vi "Init.vi"(8 "error in (no error)":errorcluster, 10 "Size":cluster{"Width":u16, "Height":u16}, 11 "Glyph Drawer in":refnum<class "Glyph Drawer.lvclass">) -> (0 "error out":errorcluster, 3 "Glyph Drawer out":refnum<class "Glyph Drawer.lvclass">)   [LabVIEW 2020, in "Glyph Drawer.lvlib" / "Glyph Drawer.lvclass"]
uses:
  Glyph Drawer.lvclass
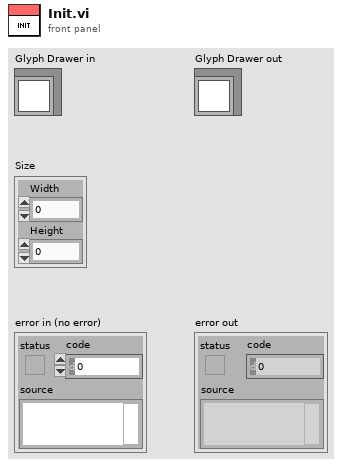
[diagram p1: front panel]
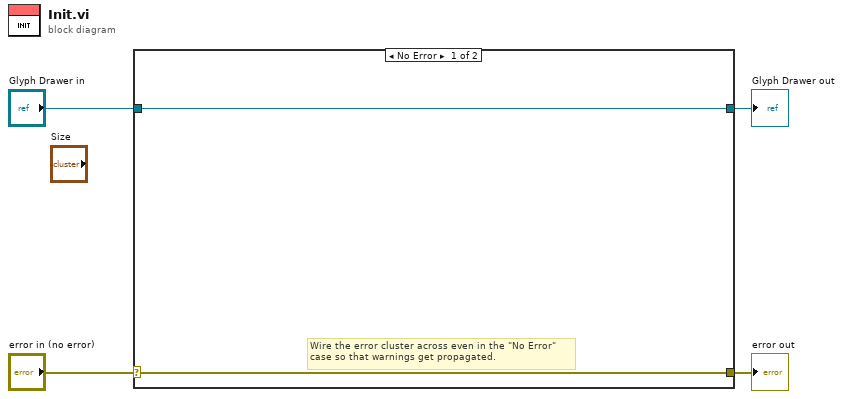
[diagram p0: block diagram]
diagram:
  n1 = case shown="No Error" "error in (no error)" {
    selector: "error in (no error)" -> [w5 w8]
    tunnel: [w5 w8] -> w3
    tunnel: [w6 w7] -> w1
    tunnel: "Glyph Drawer in" -> [w6 w7]
    frame No Error {
      # "Wire the error cluster across even in the \"No Error\"\ncase so that warnings get propagated."
    }
    frame Error {
    }
  }
  "error out" <- w3
  "Glyph Drawer out" <- w1
